vi "GLBL_9885_DO.vi"(10 "DO_8":T1, 11 "write_read":bool) -> (2 "DO_8 out":T1)   [LabVIEW 2020]
uses:
  controls/DO_0_7.ctl
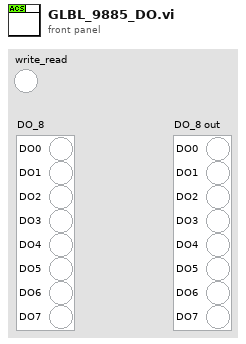
[diagram p1: front panel]
types:
  T1 = typedef "DO_0_7.ctl" = cluster{"DO0":bool, "DO1":bool, "DO2":bool, "DO3":bool, "DO4":bool, "DO5":bool, "DO6":bool, "DO7":bool}
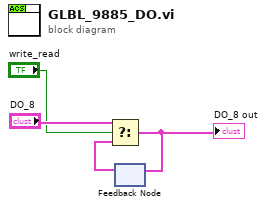
[diagram p0: block diagram]
diagram:
  n1 = feedback #1() -> (w3:T1)  [unwired: 1 in]
  n2 = Select(t="DO_8", s="write_read", f=w3) -> (s? t:f=w2:T1)
  "DO_8 out" <- w2
  n3 = feedback-in #1(w2) -> ()
